vi "Cheesy Drive.vi"(6 "Slow turn":bool, 7 "Quickturn":bool, 8 "Turn":dbl(slide) scale=-1.0..1.0, 9 "Throttle":dbl(slide) scale=-1.0..1.0) -> (1 "Right":dbl(slide) scale=-1.0..1.0, 2 "Left":dbl(slide) scale=-1.0..1.0)   [LabVIEW 2015]
uses:
  <vilib>/Rock Robotics/Network Tables/NT Read Number.vi
panel:
  in  "QT Sensitivity":dbl=0.7
  in  "QT 2":dbl=5.0
  in  "Quickturn Constant":dbl=0.1
  in  "Neg inertia constant":dbl=3.0 format="%#_13g"
  # "Outputs:"
  # "These numbers may need to be tuned"
  # "accumulation speed"
  # "maximum magnitude"
  # "Driving:\nLeft joystick: Y axis for throttle\nRight jostick: Z (twist) axis to change steering radius\n\nTrigger on right joystick activates quickturn (used to spin in place)"
  # "Driving joystick (the left one) in USB 0\nTurning joystick (the right one) in USB 1\n(change from driver station)"
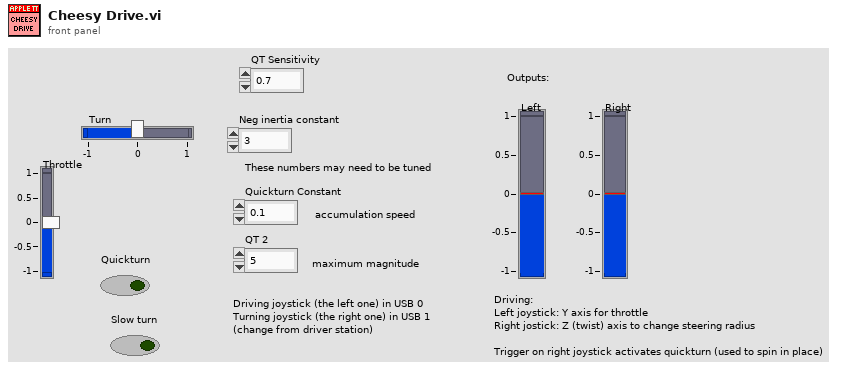
[diagram p1: front panel]
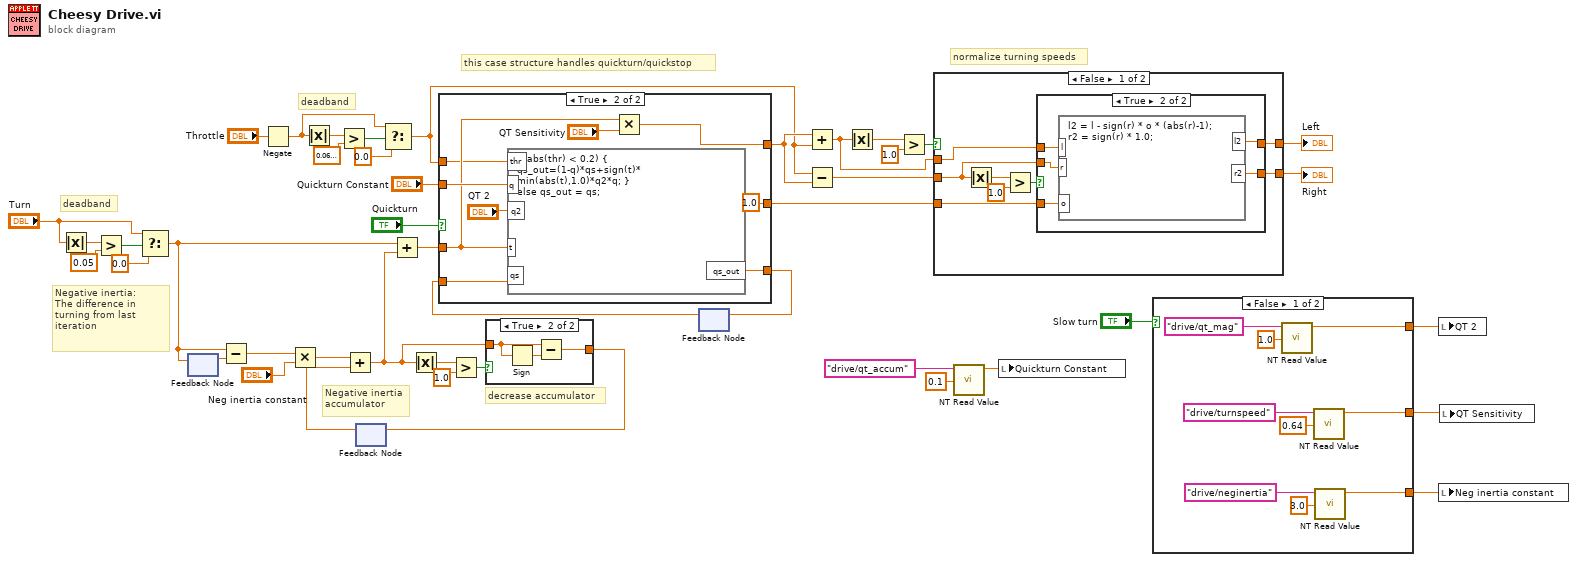
[diagram p0: block diagram]
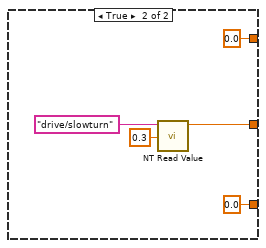
[diagram p2: hidden frame]
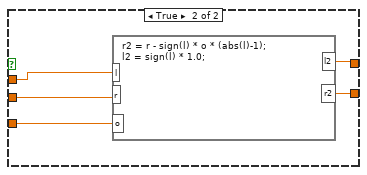
[diagram p4: hidden frame]
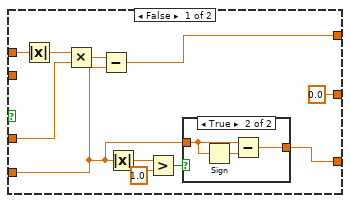
[diagram p5: hidden frame]
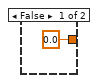
[diagram p6: hidden frame]
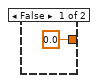
[diagram p7: hidden frame]
diagram:
  # "normalize turning speeds"
  # "this case structure handles quickturn/quickstop"
  # "deadband"
  # "deadband"
  # "decrease accumulator"
  # "Negative inertia\naccumulator"
  # "Negative inertia:\nThe difference in turning from last iteration"
  n1 = Absolute Value(x="Turn") -> (abs(x)=w14:dbl)
  n2 = Greater?(x=w14, y=0.05) -> (0:w12:bool)
  n3 = Select(t="Turn", s=w12, f=0.0) -> (s? t:f=w10:dbl)
  n4 = feedback-in #1(w10) -> ()
  n5 = feedback #1() -> (w44:dbl)  [unwired: 1 in]
  n6 = Subtract(x=w10, y=w44) -> (x-y=w43:dbl)
  n7 = Negate(x="Throttle") -> (-x=w1:dbl)
  n8 = Multiply(x=w43, y="Neg inertia constant") -> (x*y=w41:dbl)
  n9 = Absolute Value(x=w1) -> (abs(x)=w20:dbl)
  n10 = Greater?(x=w20, y=0.06999999999999999) -> (0:w18:bool)
  n11 = feedback #2() -> (w40:dbl)  [unwired: 1 in]
  n12 = Add(x=w41, y=w40) -> (x+y=w37:dbl)
  n13 = Select(t=w1, s=w18, f=0.0) -> (s? t:f=w15:dbl)
  n14 = Add(x=w10, y=w37) -> (x+y=w33:dbl)
  n15 = Absolute Value(x=w37) -> (abs(x)=w39:dbl)
  n16 = Greater?(x=w39, y=1.0) -> (0:w36:bool)
  n17 = case shown="True" w36 {
    tunnel: w37 -> [_ w47]
    tunnel: [0.0 w46] -> w30
    frame False {
    }
    frame True {
      n18 = Sign(1:w47) -> (0:w48:dbl)
      n19 = Subtract(x=w47, y=w48) -> (x-y=w46:dbl)
    }
  }
  n20 = feedback-in #2(w30) -> ()
  n21 = feedback #3() -> (w31:dbl)  [unwired: 1 in]
  n22 = case shown="True" "Quickturn" {
    tunnel: w15 -> [w50 w64]
    tunnel: "Quickturn Constant" -> [_ w72]
    tunnel: w33 -> [w58 w67]
    tunnel: w31 -> [w52 w71]
    tunnel: [w53 w70] -> w32
    tunnel: [w49 w65] -> w29
    tunnel: [0.0 1.0] -> w24
    frame False {
      n23 = Absolute Value(x=w50) -> (abs(x)=w59:dbl)
      n24 = Multiply(x=w59, y=w58) -> (x*y=w57:dbl)
      n25 = Subtract(x=w57, y=w52) -> (x-y=w49:dbl)
      n26 = Absolute Value(x=w52) -> (abs(x)=w54:dbl)
      n27 = Greater?(x=w54, y=1.0) -> (0:w56:bool)
      n28 = case shown="True" w56 {
        tunnel: w52 -> [_ w62]
        tunnel: [0.0 w61] -> w53
        frame False {
        }
        frame True {
          n29 = Sign(1:w62) -> (0:w63:dbl)
          n30 = Subtract(x=w62, y=w63) -> (x-y=w61:dbl)
        }
      }
    }
    frame True {
      # "Calculations for quickstop accumulator"
      n31 = formula code="if(abs(thr) < 0.2) {\nqs_out=(1-q)*qs+sign(t)*\nmin(abs(t),1.0)*q2*q; }\nelse qs_out = qs;"("q"=w72, "t"=w67, "qs"=w71, "q2"="QT 2", "thr"=w64) -> ("qs_out"=w70:dbl)
      n32 = Multiply(x=w67, y="QT Sensitivity") -> (x*y=w65:dbl)
    }
  }
  n33 = feedback-in #3(w32) -> ()
  n34 = Add(x=w29, y=w15) -> (x+y=w23:dbl)
  n35 = Subtract(x=w15, y=w29) -> (x-y=w25:dbl)
  n36 = Absolute Value(x=w23) -> (abs(x)=w26:dbl)
  n37 = Greater?(x=w26, y=1.0) -> (0:w28:bool)
  n38 = case shown="False" w28 {
    tunnel: [w74 w89] -> w22
    tunnel: w25 -> [w76 w91]
    tunnel: w24 -> [w75 w90]
    tunnel: w23 -> [w77 w92]
    tunnel: [w73 w88] -> w21
    frame False {
      n39 = Absolute Value(x=w76) -> (abs(x)=w80:dbl)
      n40 = Greater?(x=w80, y=1.0) -> (0:w78:bool)
      n41 = case shown="True" w78 {
        tunnel: [w82 w87] -> w74
        tunnel: [w81 w86] -> w73
        tunnel: w77 -> [w82 w85]
        tunnel: w76 -> [w81 w84]
        tunnel: w75 -> [_ w83]
        frame False {
        }
        frame True {
          n42 = formula code="l2 = l - sign(r) * o * (abs(r)-1);\nr2 = sign(r) * 1.0;"("l"=w85, "r"=w84, "o"=w83) -> ("l2"=w87:dbl, "r2"=w86:dbl)
        }
      }
    }
    frame True {
      n43 = formula code="r2 = r - sign(l) * o * (abs(l)-1);\nl2 = sign(l) * 1.0;"("l"=w92, "r"=w91, "o"=w90) -> ("l2"=w89:dbl, "r2"=w88:dbl)
    }
  }
  "Left" <- w22
  "Right" <- w21
  n44 = call-poly <vilib>:"NT Read Value.vi"("Default Value"=0.1, "Name"="drive/qt_accum") -> ("Numeric"=w6:dbl)  [unwired: 8 in, 1 out]
  n45 = local write "Quickturn Constant"(w6) -> ()
  n46 = case shown="False" "Slow turn" {
    tunnel: [w101 0.0 ("Numeric")] -> w5
    tunnel: [w96 w104] -> w4
    tunnel: [w93 0.0 ("Numeric")] -> w2
    frame False {
      n47 = call-poly <vilib>:"NT Read Value.vi"("Default Value"=1.0, "Name"="drive/qt_mag") -> ("Numeric"=w101:dbl)  [unwired: 8 in, 1 out]
      n48 = call-poly <vilib>:"NT Read Value.vi"("Default Value"=0.64, "Name"="drive/turnspeed") -> ("Numeric"=w96:dbl)  [unwired: 8 in, 1 out]
      n49 = call-poly <vilib>:"NT Read Value.vi"("Default Value"=3.0, "Name"="drive/neginertia") -> ("Numeric"=w93:dbl)  [unwired: 8 in, 1 out]
    }
    frame True {
      n50 = call-poly <vilib>:"NT Read Value.vi"("Default Value"=0.3, "Name"="drive/slowturn") -> ("Numeric"=w104:dbl)  [unwired: 8 in, 1 out]
    }
  }
  n51 = local write "QT 2"(w5) -> ()
  n52 = local write "Neg inertia constant"(w2) -> ()
  n53 = local write "QT Sensitivity"(w4) -> ()
